vi "FTW-STR-Indent.vi"(2 "Skip first line?":bool, 5 "String":string, 7 "Indentation Characters":string="    ") -> (6 "Indented String":string)   [LabVIEW 2015]
panel:
  # "Inputs"
  # "Outputs"
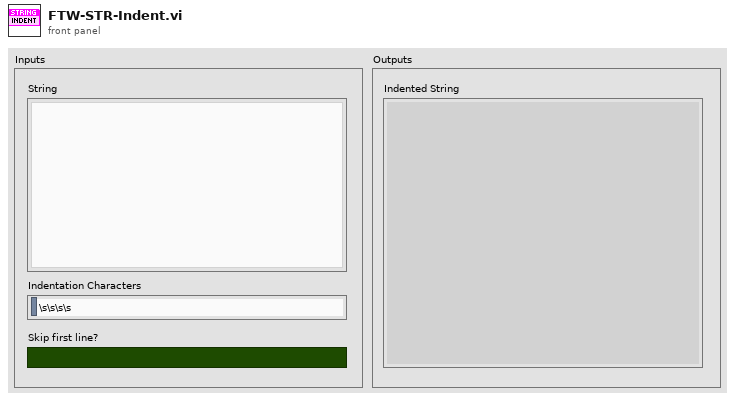
[diagram p1: front panel]
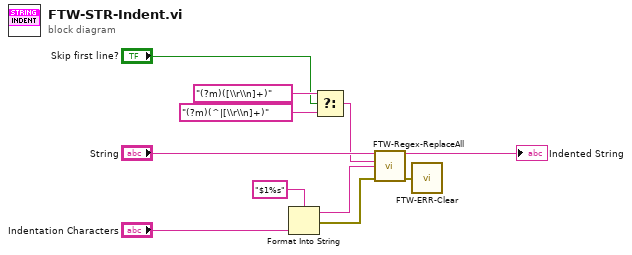
[diagram p0: block diagram]
diagram:
  n1 = Format Into String(format string="$1%s", "Indentation Characters") -> (resulting string=w7:string, error out=w5:errorcluster)  [unwired: 2 in]
  n2 = Select(t="(?m)([\\r\\n]+)", s="Skip first line?", f="(?m)(^|[\\r\\n]+)") -> (s? t:f=w2:string)
  n3 = call "FTW-Regex-ReplaceAll.vi"("String"="String", "Search for (Regular Expression)"=w2, "Replace with"=w7, "error in"=w5) -> ("String out"=→"Indented String":string, "error out"=w6:errorcluster)  [unwired: 9 in, 1 out]
  n4 = call "FTW-ERR-Clear.vi"("error to snuff"=w6) -> ()  [unwired: 1 out]
